vi "Read Memory.vi"(0 "connection ID":refnum<k16>, 1 "address":u32, 2 "port":u16, 5 "Memory Address":u16, 9 "timeout ms (1000)":i32=1000, 11 "error in (no error)":errorcluster) -> (4 "connection ID out":refnum<k16>, 6 "received data":string, 8 "Memory Data":i16, 15 "error out":errorcluster)   [LabVIEW 2016, in "instr.lvlib"]
doc: "Reads given memory item."
uses:
  instr.lvlib
panel:
  out "Send String":string
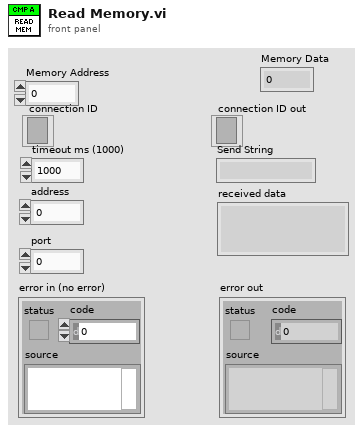
[diagram p1: front panel]
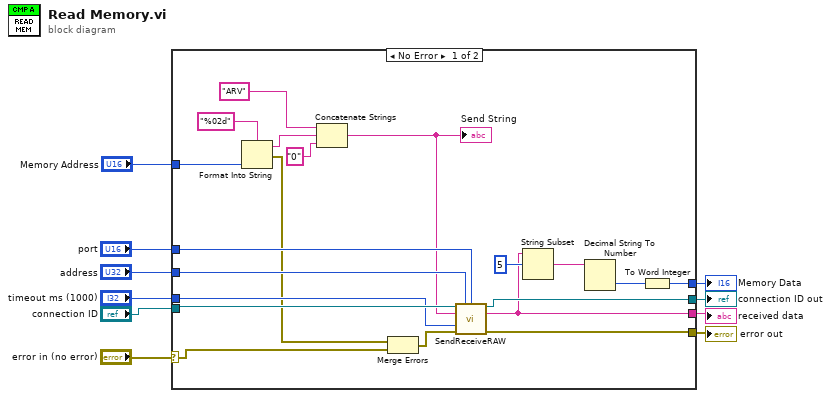
[diagram p0: block diagram]
diagram:
  n1 = case shown="No Error" "error in (no error)" {
    selector: "error in (no error)" -> [w18 w32]
    tunnel: [w30 w32] -> w10
    tunnel: "timeout ms (1000)" -> [w27 _]
    tunnel: "connection ID" -> [w28 w31]
    tunnel: [w29 w31] -> w6
    tunnel: "address" -> [w26 _]
    tunnel: "port" -> [w25 _]
    tunnel: [w23 _] -> w3
    tunnel: "Memory Address" -> [w19 _]
    tunnel: [w12 _] -> w1
    frame No Error {
      n2 = Format Into String(format string="%02d", w19) -> (resulting string=w20:string, error out=w15:errorcluster)  [unwired: 2 in]
      n3 = Concatenate Strings("ARV" ("data in"), w20, "0" ("string")) -> (w16:string)
      "Send String" <- w16
      n4 = Merge Errors(w15, w18) -> (w14:errorcluster)
      n5 = call "SendReceiveRAW.vi"("connection ID"=w28, "address"=w26, "port"=w25, "RAW data in"=w16, "timeout ms (1000)"=w27, "error in (no error)"=w14) -> ("connection ID out"=w29:refnum<k16>, "received data"=w23:string, "error out"=w30:errorcluster)  [unwired: 7 in]
      n6 = String Subset(string=w23, offset (0)=5 ("offset")) -> (substring=w13:string)  [unwired: 1 in]
      n7 = Decimal String To Number(string=w13) -> (number=w11:i32)  [unwired: 2 in, 1 out]
      n8 = To Word Integer(number=w11) -> (16bit integer=w12:i16)
    }
    frame Error {
    }
  }
  "error out" <- w10
  "received data" <- w3
  "connection ID out" <- w6
  "Memory Data" <- w1
